vi "RSZVB Trace Stimulus Data ZVR.vi"(8 "error in (no error)":errorcluster {"code" format="%.0x"}, 10 "Data Format (0: Channel 1 Data)":i32(ring) items=["Channel 1 Data", "Channel 2 Data", "Channel 3 Data", "Channel 4 Data", "Channel 1 Memory", "Channel 2 Memory", "Channel 3 Memory", "Channel 4 Memory", "Memory Trace 1", "Memory Trace 2", "Memory Trace 3", "Memory Trace 4", "Memory Trace 5", "Memory Trace 6", "Memory Trace 7", "Memory Trace 8"], 11 "VISA session":refnum<visa-resource-name>) -> (0 "error out":errorcluster {"code" format="%.0x"}, 2 "Trace Data":dbl[](array[numeric]) format="%^.3e", 3 "dup VISA session":refnum<visa-resource-name>)   [LabVIEW 2011]
doc: "This VI returns the stimulus values of the active data trace or memory trace.\n\nNote(s):\n\n(1) This VI is ZVR compatible.\n\nRemote-control command(s):\nFORMat[:DATA] REAL ,32\nTRACe[:DATA]:STIMulus[:ALL]? CH1DATA | CH2DATA | CH3DATA | CH4DATA | CH1MEM | CH2MEM | CH3MEM | CH4MEM | MDATA1 | MDATA2 | MDATA3 | MDATA4 | MDATA5 | MDATA6 | MDATA7 | MDATA8"
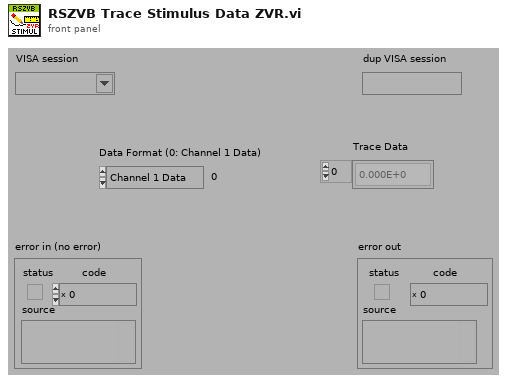
[diagram p1: front panel]
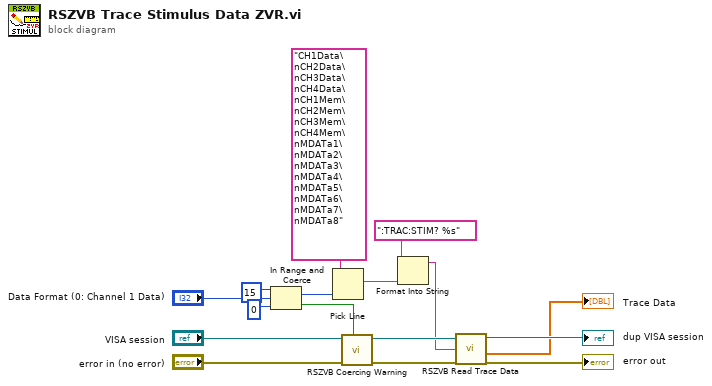
[diagram p0: block diagram]
diagram:
  n1 = In Range and Coerce(upper limit=15, x="Data Format (0: Channel 1 Data)", lower limit=0) -> (coerced(x)=w13:i32, In Range?=w11:bool)
  n2 = Pick Line(multi-line string="CH1Data\nCH2Data\nCH3Data\nCH4Data\nCH1Mem\nCH2Mem\nCH3Mem\nCH4Mem\nMDATa1\nMDATa2\nMDATa3\nMDATa4\nMDATa5\nMDATa6\nMDATa7\nMDATa8", line index=w13) -> (output string=w10:string)  [unwired: 1 in]
  n3 = call "RSZVB Coercing Warning.vi"("In Range?"=w11, "error in (no error)"="error in (no error)", "VISA session"="VISA session") -> ("error out"=w5:errorcluster, "dup VISA session"=w6:refnum<visa-resource-name>)  [unwired: 7 in]
  n4 = Format Into String(format string=":TRAC:STIM? %s", w10) -> (resulting string=w4:string)  [unwired: 2 in, 1 out]
  n5 = call "RSZVB Read Trace Data.vi"("error in (no error)"=w5, "Buffer"=w4, "VISA session"=w6) -> ("error out"=→"error out":errorcluster, "Trace Data"=→"Trace Data":dbl[], "dup VISA session"=→"dup VISA session":refnum<visa-resource-name>)  [unwired: 6 in]
